vi "OLA.vi"() -> ()   [LabVIEW 2009]
doc: "This is the On-Line Analysis module (OLA).\nThis module receives events from the Target Event Builder (TEB) and processes them. The Q Curve is massaged, gains are divided out, the subtracted and poly subtracted signals are calculated, and an area measurement is made. These results are then sent to the Polarization Display Panel (PDP)."
uses:
  <vilib>/Analysis/NI_AALPro.lvlib
  <vilib>/Analysis/NI_AALBase.lvlib
panel:
  out "Bottom Charge":dbl format="%.6e"
  out "Top Charge":dbl format="%.6e"
  in  "Previous Event":i32
  in  "stop":bool
  out "RF Mod":i32
  out "RF Freq":dbl format="%.3f"
  out "Cal Const":dbl format="%.6f"
  out "Baseline":i32
  out "Raw Signal":dbl[](array[numeric]) format="%.4f"
  out "Event Number":i32
  out "Area":dbl format="%.6f"
  out "Polarization":dbl format="%.2f"
  out "PolySubtracted Signal":dbl[](array[numeric]) format="%.4f"
  out "Polyfit Curve":dbl[](array[numeric]) format="%.4f"
  out "Subtracted Signal":dbl[](array[numeric]) format="%.4f"
  out "Baseline Signal":dbl[](array[numeric]) format="%.6f"
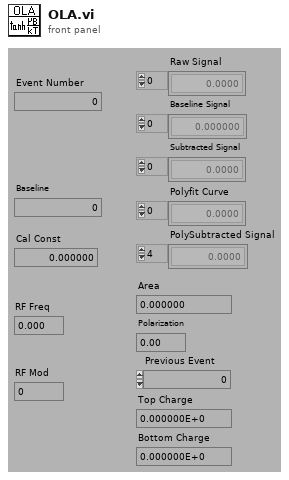
[diagram p1: front panel]
types:
  T1 = enum32{"SVD", "Givens", "Givens2", "Householder", "LU Decomposition", "Cholesky"}
  T2 = enum16{"No Message", "Bad Message", "ClearCharge", "Event=", "Address=", "Ping=", "Stop"}
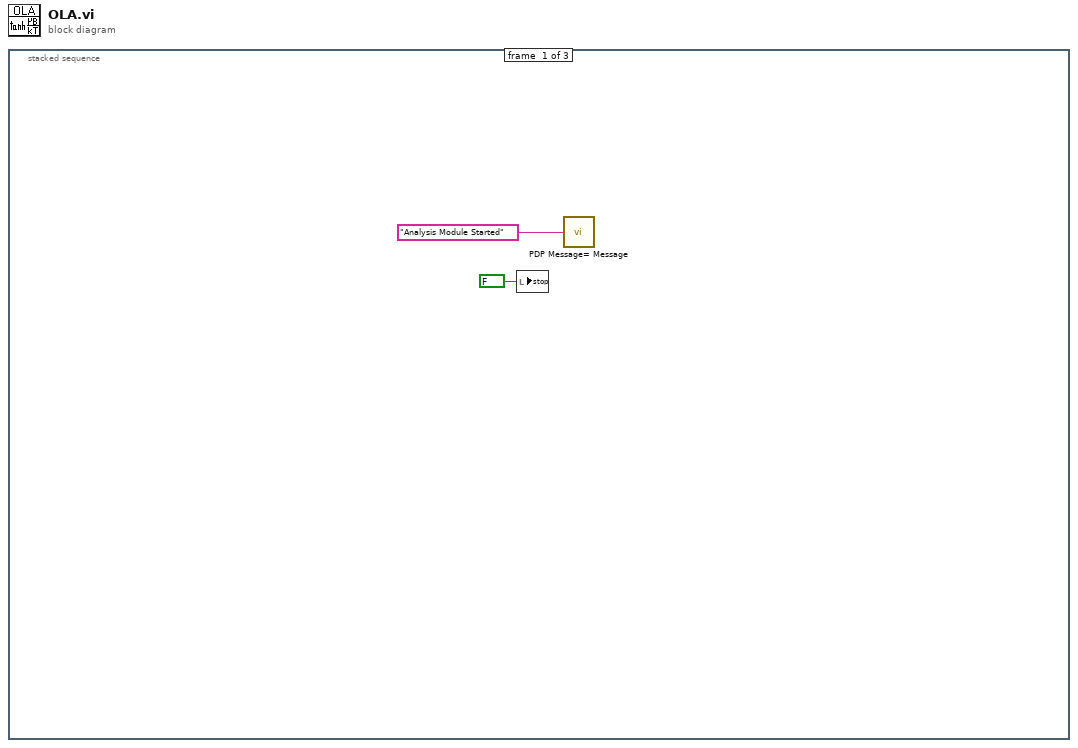
[diagram p0: block diagram]
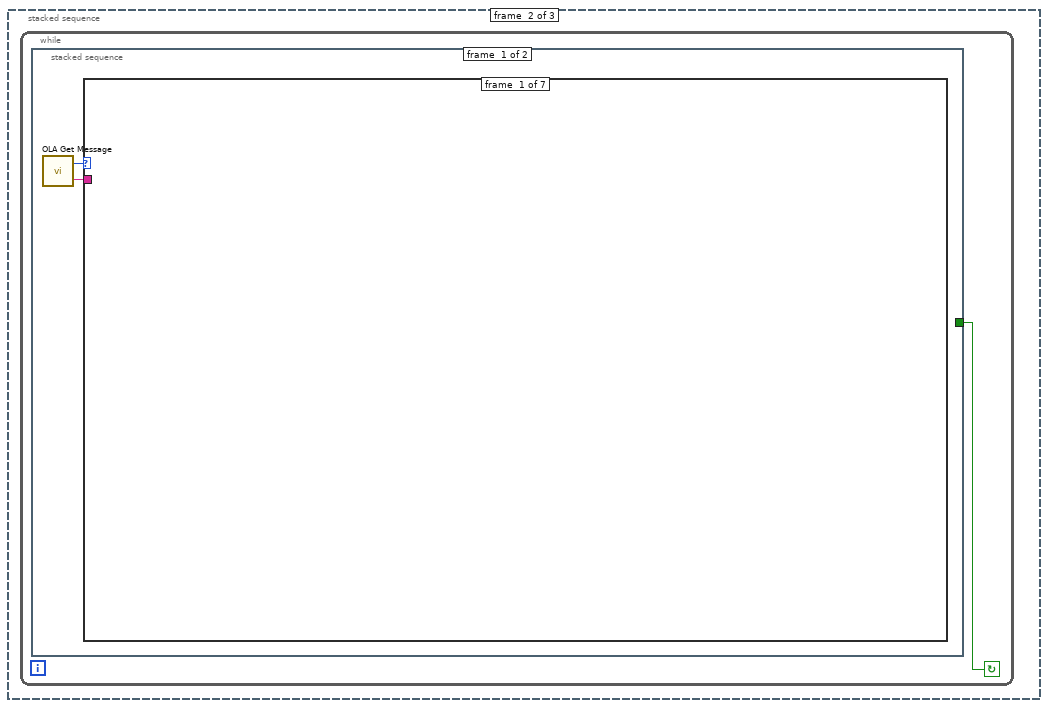
[diagram p2: hidden frame]
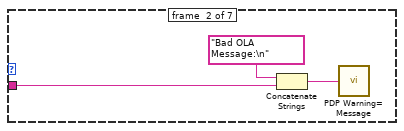
[diagram p3: hidden frame]
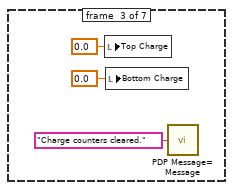
[diagram p4: hidden frame]
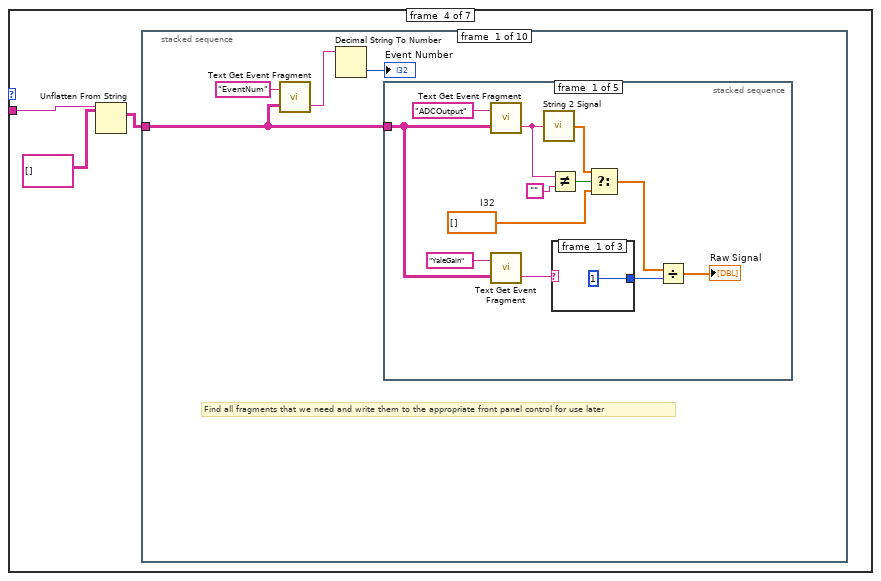
[diagram p5: hidden frame]
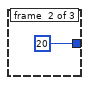
[diagram p6: hidden frame]
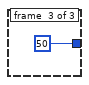
[diagram p7: hidden frame]
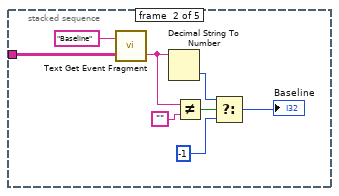
[diagram p8: hidden frame]
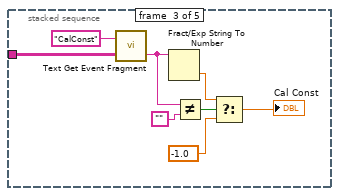
[diagram p9: hidden frame]
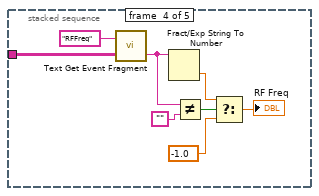
[diagram p10: hidden frame]
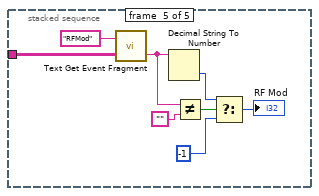
[diagram p11: hidden frame]
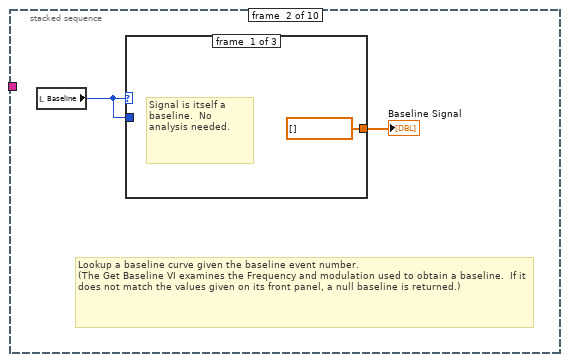
[diagram p12: hidden frame]
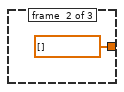
[diagram p13: hidden frame]
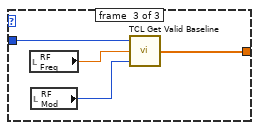
[diagram p14: hidden frame]
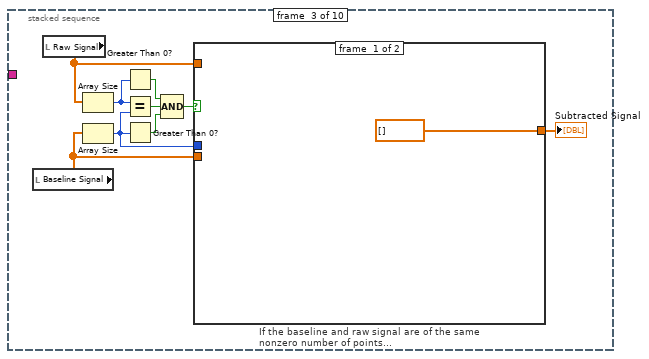
[diagram p15: hidden frame]
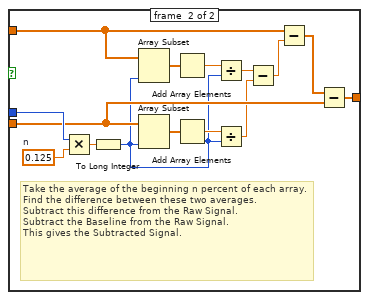
[diagram p16: hidden frame]
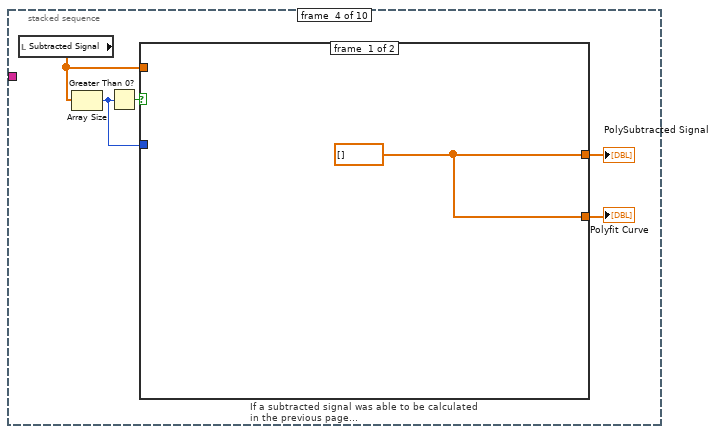
[diagram p17: hidden frame]
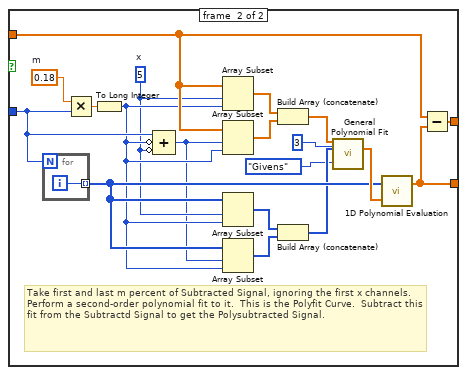
[diagram p18: hidden frame]
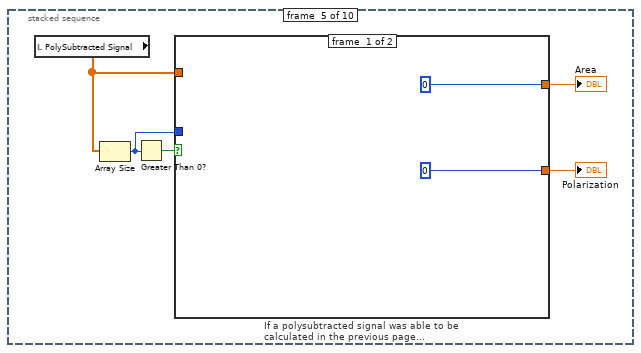
[diagram p19: hidden frame]
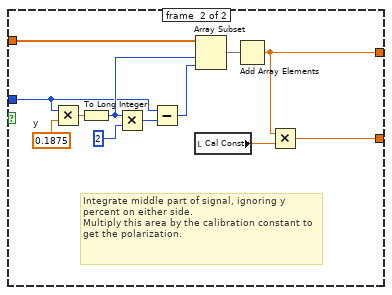
[diagram p20: hidden frame]
diagram:
  n1 = stacked-sequence {
    frame #0 {
      n2 = local write "stop"(FALSE ("stop")) -> ()
      n3 = call "PDP Message= Message.vi"("Message"="Analysis Module Started") -> ()
    }
    frame #1 {
      n4 = while {
        stop <- w3 continue-if-true
        n5 = stacked-sequence {
          tunnel: [_ w282] -> w3
          frame #0 {
            n6 = call "OLA Get Message.vi"() -> ("Text"=w5:string, "OLA Message Type"=w4:T2)
            n7 = case shown="\"Event=\"" w4 {
              tunnel: w5 -> [_ w8 _ w13 w274 w277 _]
              frame #0 {
              }
              frame #1 {
                n8 = Concatenate Strings("Bad OLA Message:\n", w8) -> (w6:string)
                n9 = call "PDP Warning= Message.vi"("Message"=w6) -> ()
              }
              frame #2 {
                n10 = local write "Top Charge"(0.0 ("Top Charge")) -> ()
                n11 = local write "Bottom Charge"(0.0 ("Bottom Charge")) -> ()
                n12 = call "PDP Message= Message.vi"("Message"="Charge counters cleared.") -> ()
              }
              frame #3 {
                (unwired) FALSE
                n13 = Unflatten From String(type=string[][] [], binary string=w13) -> (value=w12:string[][])  [unwired: 3 in, 2 out]
                n14 = stacked-sequence {
                  tunnel: w12 -> [w15 _ _ _ _ w147 w180 w199 _ _]
                  frame #0 {
                    # "Find all fragments that we need and write them to the appropriate front panel control for use later"
                    n15 = call "Text Get Event Fragment.vi"("Event"=w15, "Fragment Type"="EventNum") -> ("Fragment"=w17:string)  [unwired: 1 out]
                    n16 = Decimal String To Number(string=w17) -> (number=→"Event Number":i32)  [unwired: 2 in, 1 out]
                    n17 = stacked-sequence {
                      tunnel: w15 -> [w24 w40 w48 w56 w64]
                      frame #0 {
                        w19 = dbl[] []  # I32
                        n18 = call "Text Get Event Fragment.vi"("Event"=w24, "Fragment Type"="ADCOutput") -> ("Fragment"=w29:string)  [unwired: 1 out]
                        n19 = call "Text Get Event Fragment.vi"("Event"=w24, "Fragment Type"="YaleGain") -> ("Fragment"=w23:string)  [unwired: 1 out]
                        n20 = call "String 2 Signal.vi"("String"=w29) -> ("Signal"=w26:dbl[])
                        n21 = Not Equal?(x=w29, y="") -> (x != y?=w28:bool)
                        n22 = case shown="\"2\"" w23 {
                          tunnel: [1 20 50] -> w22
                          frame #0 {
                          }
                          frame #1 {
                          }
                          frame #2 {
                          }
                        }
                        n23 = Select(t=w26, s=w28, f=w19) -> (s? t:f=w21:dbl[])
                        n24 = Divide(x=w21, y=w22) -> (x/y=→"Raw Signal":dbl[])
                      }
                      frame #1 {
                        n25 = call "Text Get Event Fragment.vi"("Event"=w40, "Fragment Type"="Baseline") -> ("Fragment"=w35:string)  [unwired: 1 out]
                        n26 = Decimal String To Number(string=w35) -> (number=w38:i32)  [unwired: 2 in, 1 out]
                        n27 = Not Equal?(x=w35, y="") -> (x != y?=w37:bool)
                        n28 = Select(t=w38, s=w37, f=-1) -> (s? t:f=→"Baseline":i32)
                      }
                      frame #2 {
                        n29 = call "Text Get Event Fragment.vi"("Event"=w48, "Fragment Type"="CalConst") -> ("Fragment"=w43:string)  [unwired: 1 out]
                        n30 = Fract/Exp String To Number(string=w43) -> (number=w46:dbl)  [unwired: 3 in, 1 out]
                        n31 = Not Equal?(x=w43, y="") -> (x != y?=w45:bool)
                        n32 = Select(t=w46, s=w45, f=-1.0) -> (s? t:f=→"Cal Const":dbl)
                      }
                      frame #3 {
                        n33 = call "Text Get Event Fragment.vi"("Event"=w56, "Fragment Type"="RFFreq") -> ("Fragment"=w51:string)  [unwired: 1 out]
                        n34 = Fract/Exp String To Number(string=w51) -> (number=w54:dbl)  [unwired: 3 in, 1 out]
                        n35 = Not Equal?(x=w51, y="") -> (x != y?=w53:bool)
                        n36 = Select(t=w54, s=w53, f=-1.0) -> (s? t:f=→"RF Freq":dbl)
                      }
                      frame #4 {
                        n37 = call "Text Get Event Fragment.vi"("Event"=w64, "Fragment Type"="RFMod") -> ("Fragment"=w59:string)  [unwired: 1 out]
                        n38 = Decimal String To Number(string=w59) -> (number=w62:i32)  [unwired: 2 in, 1 out]
                        n39 = Not Equal?(x=w59, y="") -> (x != y?=w61:bool)
                        n40 = Select(t=w62, s=w61, f=-1) -> (s? t:f=→"RF Mod":i32)
                      }
                    }
                  }
                  frame #1 {
                    # "Lookup a baseline curve given the baseline event number.\n(The Get Baseline VI examines the Frequency and modulation used to obtain a baseline.  If it does not match the values given on its front panel, a null baseline is returned.)"
                    n41 = local read "Baseline"() -> (w67:i32)
                    n42 = case shown="1, Default" w67 {
                      tunnel: w67 -> [_ _ w73]
                      tunnel: [dbl[] [] ("Baseline") dbl[] [] ("Baseline") w70] -> w66
                      frame #0 {
                        # "Signal is itself a baseline.  No analysis needed."
                      }
                      frame #1 {
                      }
                      frame #2 {
                        n43 = local read "RF Freq"() -> (w72:dbl)
                        n44 = local read "RF Mod"() -> (w71:i32)
                        n45 = call "TCL Get Valid Baseline.vi"("RFMod (kHz)"=w71, "RFFreq (MHz)"=w72, "Baseline Event #"=w73) -> ("Baseline"=w70:dbl[])
                      }
                    }
                    "Baseline Signal" <- w66
                  }
                  frame #2 {
                    n46 = local read "Baseline Signal"() -> (w82:dbl[])
                    n47 = local read "Raw Signal"() -> (w81:dbl[])
                    n48 = Array Size(array=w81) -> (size(s)=w79:i32)
                    n49 = Array Size(array=w82) -> (size(s)=w80:i32)
                    n50 = Greater Than 0?(x=w79) -> (x > 0?=w76:bool)
                    n51 = Equal?(x=w79, y=w80) -> (x = y?=w77:bool)
                    n52 = Greater Than 0?(x=w80) -> (x > 0?=w78:bool)
                    n53 = Compound Arithmetic op=AND(w76, w77, w78) -> (w75:bool)
                    n54 = case "If the baseline and raw signal are of the same nonzero number of points..." shown="True" w75 {
                      tunnel: w82 -> [_ w91]
                      tunnel: w81 -> [_ w93]
                      tunnel: w80 -> [_ w98]
                      tunnel: [dbl[] [] w84] -> w74
                      frame #0 {
                      }
                      frame #1 {
                        w96 = 0.125  # n
                        # "Take the average of the beginning n percent of each array.\nFind the difference between these two averages.\nSubtract this difference from the Raw Signal.\nSubtract the Baseline from the Raw Signal.\nThis gives the Subtracted Signal."
                        n55 = Multiply(x=w98, y=w96) -> (x*y=w97:dbl)
                        n56 = To Long Integer(number=w97) -> (32bit integer=w85:i32)
                        n57 = Array Subset(array=w93, length=w85) -> (w95:dbl[])  [unwired: 1 in]
                        n58 = Array Subset(array=w91, length=w85) -> (w94:dbl[])  [unwired: 1 in]
                        n59 = Add Array Elements(numeric array=w95) -> (sum=w89:dbl)
                        n60 = Add Array Elements(numeric array=w94) -> (sum=w90:dbl)
                        n61 = Divide(x=w89, y=w85) -> (x/y=w88:dbl)
                        n62 = Divide(x=w90, y=w85) -> (x/y=w87:dbl)
                        n63 = Subtract(x=w88, y=w87) -> (x-y=w86:dbl)
                        n64 = Subtract(x=w93, y=w86) -> (x-y=w92:dbl[])
                        n65 = Subtract(x=w92, y=w91) -> (x-y=w84:dbl[])
                      }
                    }
                    "Subtracted Signal" <- w74
                  }
                  frame #3 {
                    n66 = local read "Subtracted Signal"() -> (w101:dbl[])
                    n67 = Array Size(array=w101) -> (size(s)=w102:i32)
                    n68 = Greater Than 0?(x=w102) -> (x > 0?=w103:bool)
                    n69 = case "If a subtracted signal was able to be calculated in the previous page..." shown="True" w103 {
                      tunnel: w102 -> [_ w108]
                      tunnel: w101 -> [_ w111]
                      tunnel: [w104 w110] -> w100
                      tunnel: [w104 w109] -> w99
                      frame #0 {
                        w104 = dbl[] []
                      }
                      frame #1 {
                        w106 = 5  # x
                        w123 = 0.18  # m
                        # "Take first and last m percent of Subtracted Signal, ignoring the first x channels.  Perform a second-order polynomial fit to it.  This is the Polyfit Curve.  Subtract this fit from the Subtractd Signal to get the Polysubtracted Signal."
                        n70 = for {
                          N: w108 -> [_]
                          tunnel: [w124] -> w116 mode=indexing
                          i -> [w124]
                        }
                        n71 = Multiply(x=w123, y=w108) -> (x*y=w122:dbl)
                        n72 = To Long Integer(number=w122) -> (32bit integer=w107:i32)
                        n73 = Compound Arithmetic op=ADD(w108, invert w107, invert w106) -> (w105:i32)
                        n74 = Array Subset(array=w111, index=w106, length=w107) -> (w121:dbl[])
                        n75 = Array Subset(array=w111, index=w105, length=w107) -> (w120:dbl[])
                        n76 = Array Subset(array=w116, index=w106, length=w107) -> (w119:i32[])
                        n77 = Array Subset(array=w116, index=w105, length=w107) -> (w118:i32[])
                        n78 = Build Array (concatenate)(w121, w120) -> (w115:dbl[])
                        n79 = Build Array (concatenate)(w119, w118) -> (w114:i32[])
                        n80 = call <vilib>:"General Polynomial Fit.vi"("Y"=w115, "polynomial order"=3, "X"=w114, "algorithm"=T1."Givens") -> ("Polynomial Coefficients"=w117:dbl[])  [unwired: 8 in, 3 out]
                        n81 = call <vilib>:"1D Polynomial Evaluation.vi"("Coefficients: a"=w117, "X"=w116) -> ("Y"=w109:dbl[])  [unwired: 1 out]
                        n82 = Subtract(x=w111, y=w109) -> (x-y=w110:dbl[])
                      }
                    }
                    "Polyfit Curve" <- w99
                    "PolySubtracted Signal" <- w100
                  }
                  frame #4 {
                    n83 = local read "PolySubtracted Signal"() -> (w128:dbl[])
                    n84 = Array Size(array=w128) -> (size(s)=w127:i32)
                    n85 = Greater Than 0?(x=w127) -> (x > 0?=w129:bool)
                    n86 = case "If a polysubtracted signal was able to be calculated in the previous page..." shown="True" w129 {
                      tunnel: w128 -> [_ w143]
                      tunnel: w127 -> [_ w135]
                      tunnel: [0 w134] -> w126
                      tunnel: [0 w133] -> w125
                      frame #0 {
                      }
                      frame #1 {
                        w141 = 0.1875  # y
                        # "Integrate middle part of signal, ignoring y percent on either side.\nMultiply this area by the calibration constant to get the polarization."
                        n87 = Multiply(x=w135, y=w141) -> (x*y=w139:dbl)
                        n88 = To Long Integer(number=w139) -> (32bit integer=w136:i32)
                        n89 = Multiply(x=w136, y=2) -> (x*y=w137:i32)
                        n90 = Subtract(x=w135, y=w137) -> (x-y=w140:i32)
                        n91 = local read "Cal Const"() -> (w132:dbl)
                        n92 = Array Subset(array=w143, index=w136, length=w140) -> (w142:dbl[])
                        n93 = Add Array Elements(numeric array=w142) -> (sum=w134:dbl)
                        n94 = Multiply(x=w134, y=w132) -> (x*y=w133:dbl)
                      }
                    }
                    "Polarization" <- w125
                    "Area" <- w126
                  }
                  frame #5 {
                    n95 = call "Text Get Event Fragment.vi"("Event"=w147, "Fragment Type"="ptpos") -> ("Fragment"=w145:string)  [unwired: 1 out]
                    n96 = call "Text Get Event Fragment.vi"("Event"=w147, "Fragment Type"="ibcm2") -> ("Fragment"=w156:string, "Found"=w144:bool)
                    n97 = call "Text Get Event Fragment.vi"("Event"=w147, "Fragment Type"="LL91112") -> ("Fragment"=w158:string)  [unwired: 1 out]
                    n98 = Fract/Exp String To Number(string=w156) -> (number=w155:dbl)  [unwired: 3 in, 1 out]
                    n99 = Fract/Exp String To Number(string=w158) -> (number=w157:dbl)  [unwired: 3 in, 1 out]
                    n100 = Greater?(x=w155, y=20.0) -> (0:w150:bool)
                    n101 = Less?(x=w155, y=200.0) -> (x < y?=w152:bool)
                    n102 = Not Equal To 0?(x=w157) -> (x != 0?=w151:bool)
                    n103 = Compound Arithmetic op=AND(w144, w150, w152, w151) -> (w149:bool)
                    n104 = case shown="True" w149 {
                      tunnel: w155 -> [_ w170]
                      tunnel: w145 -> [_ w161]
                      frame #0 {
                      }
                      frame #1 {
                        w169 = 100  # n
                        # "Only add to charge if less than n seconds since last event"
                        n105 = local read "Event Number"() -> (w160:i32)
                        n106 = Subtract(x=w160, y="Previous Event") -> (x-y=w166:i32)
                        n107 = case shown="\"1\"" w161 {
                          tunnel: [0.0 w177 w178] -> w163
                          frame #0 {
                          }
                          frame #1 {
                            n108 = local read "Top Charge"() -> (w177:dbl)
                          }
                          frame #2 {
                            n109 = local read "Bottom Charge"() -> (w178:dbl)
                          }
                        }
                        n110 = Less?(x=w166, y=w169) -> (x < y?=w167:bool)
                        n111 = Select(t=w166, s=w167, f=0) -> (s? t:f=w164:i32)
                        n112 = Compound Arithmetic op=MULTIPLY(w170, 6.241418050181001e+18, 1e-09 ("Input"), w164) -> (w168:dbl)
                        n113 = Add(x=w163, y=w168) -> (x+y=w162:dbl)
                        n114 = local write "Previous Event"(w160) -> ()
                        n115 = case shown="\"1\"" w161 {
                          tunnel: w162 -> [_ w174 w175]
                          frame #0 {
                          }
                          frame #1 {
                            "Top Charge" <- w174
                          }
                          frame #2 {
                            "Bottom Charge" <- w175
                          }
                        }
                      }
                    }
                  }
                  frame #6 {
                    n116 = call "Text Get Event Fragment.vi"("Event"=w180, "Fragment Type"="He4Temp") -> ("Found"=w179:bool)  [unwired: 1 out]
                    n117 = case shown="False" w179 {
                      tunnel: w180 -> [w188 _]
                      frame #0 {
                        n118 = call "Text Get Event Fragment.vi"("Event"=w188, "Fragment Type"="He4Press") -> ("Fragment"=w196:string)  [unwired: 1 out]
                        n119 = call "Text Get Event Fragment.vi"("Event"=w188, "Fragment Type"="He4Range") -> ("Fragment"=w187:string)  [unwired: 1 out]
                        n120 = Fract/Exp String To Number(string=w196) -> (number=w182:dbl)  [unwired: 3 in, 1 out]
                        n121 = Fract/Exp String To Number(string=w187) -> (number=w186:dbl)  [unwired: 3 in, 1 out]
                        n122 = expression code="10**(-x+2)"(w186) -> (w185:dbl)
                        n123 = Multiply(x=w182, y=w185) -> (x*y=w183:dbl)
                        n124 = call "TTM 4He Press to Temp.vi"("4He Vapor Pressure (torr)"=w183) -> ("4He Temp (K)"=w184:dbl)
                        n125 = Number To Exponential String(number=w184) -> (E-format string=w194:string)  [unwired: 3 in]
                        n126 = local read "Event Number"() -> (w191:i32)
                        n127 = Build Array("He4Temp", w194) -> (w190:string[])
                        n128 = Build Array(w190) -> (w192:string[][])
                        n129 = call "TEB EventFrag= Message.vi"("Event Fragment(s)"=w192, "Event Number"=w191) -> ()
                      }
                      frame #1 {
                      }
                    }
                  }
                  frame #7 {
                    n130 = call "Text Get Event Fragment.vi"("Event"=w199, "Fragment Type"="HPFreq") -> ("Fragment"=w197:string, "Found"=w198:bool)
                    n131 = case shown="True" w198 {
                      tunnel: w199 -> [w202 w220]
                      tunnel: w197 -> [_ w217]
                      frame #0 {
                        n132 = call "Text Get Event Fragment.vi"("Event"=w202, "Fragment Type"="EIPFreq") -> ("Fragment"=w201:string)  [unwired: 1 out]
                        n133 = local read "Event Number"() -> (w204:i32)
                        n134 = Build Array("uWaveFreq", w201) -> (w203:string[])
                        n135 = Build Array(w203) -> (w205:string[][])
                        n136 = call "TEB EventFrag= Message.vi"("Event Fragment(s)"=w205, "Event Number"=w204) -> ()
                      }
                      frame #1 {
                        n137 = call "Text Get Event Fragment.vi"("Event"=w220, "Fragment Type"="EIPFreq") -> ("Fragment"=w219:string)  [unwired: 1 out]
                        n138 = Fract/Exp String To Number(string=w217) -> (number=w210:dbl)  [unwired: 3 in, 1 out]
                        n139 = Fract/Exp String To Number(string=w219) -> (number=w218:dbl)  [unwired: 3 in, 1 out]
                        n140 = Multiply(x=w218, y=2) -> (x*y=w216:dbl)
                        n141 = Add(x=w210, y=w216) -> (x+y=w215:dbl)
                        n142 = Equal To 0?(x=w210) -> (x = 0?=w209:bool)
                        n143 = Number To Fractional String(number=w215, precision (6)=i16 3) -> (F-format string=w211:string)  [unwired: 2 in]
                        n144 = Select(t="0", s=w209, f=w211) -> (s? t:f=w212:string)
                        n145 = local read "Event Number"() -> (w222:i32)
                        n146 = Build Array("uWaveFreq", w212) -> (w221:string[])
                        n147 = Build Array(w221) -> (w223:string[][])
                        n148 = call "TEB EventFrag= Message.vi"("Event Fragment(s)"=w223, "Event Number"=w222) -> ()
                      }
                    }
                  }
                  frame #8 {
                    w228 = string[] [] ("Array Constant")
                    # "Ship all results off to the event builder."
                    n149 = local read "PolySubtracted Signal"() -> (w226:dbl[])
                    n150 = local read "Polyfit Curve"() -> (w262:dbl[])
                    n151 = local read "Bottom Charge"() -> (w238:dbl)
                    n152 = local read "Subtracted Signal"() -> (w263:dbl[])
                    n153 = local read "Top Charge"() -> (w239:dbl)
                    n154 = local read "Polarization"() -> (w249:dbl)
                    n155 = local read "Raw Signal"() -> (w246:dbl[])
                    n156 = local read "Baseline Signal"() -> (w268:dbl[])
                    n157 = local read "Area"() -> (w257:dbl)
                    n158 = Array Size(array=w226) -> (size(s)=w227:i32)
                    n159 = Equal To 0?(x=w227) -> (x = 0?=w229:bool)
                    n160 = call "Signal 2 String.vi"("Signal"=w246) -> ("String"=w247:string)
                    n161 = call "Signal 2 String.vi"("Signal"=w268) -> ("String"=w267:string)
                    n162 = call "Signal 2 String.vi"("Signal"=w263) -> ("String"=w264:string)
                    n163 = call "Signal 2 String.vi"("Signal"=w262) -> ("String"=w261:string)
                    n164 = call "Signal 2 String.vi"("Signal"=w226) -> ("String"=w258:string)
                    n165 = Number To Exponential String(number=w239) -> (E-format string=w241:string)  [unwired: 3 in]
                    n166 = Number To Exponential String(number=w238) -> (E-format string=w236:string)  [unwired: 3 in]
                    n167 = Number To Exponential String(number=w249) -> (E-format string=w250:string)  [unwired: 3 in]
                    n168 = Number To Exponential String(number=w257) -> (E-format string=w256:string)  [unwired: 3 in]
                    n169 = Build Array("RawSignal", w247) -> (w245:string[])
                    n170 = Build Array("BaseSignal", w267) -> (w244:string[])
                    n171 = Build Array("SubSignal", w264) -> (w243:string[])
                    n172 = Build Array("PolyCurve", w261) -> (w242:string[])
                    n173 = Build Array("PolySignal", w258) -> (w254:string[])
                    n174 = Build Array("TopCharge", w241) -> (w235:string[])
                    n175 = Build Array("BottomCharge", w236) -> (w234:string[])
                    n176 = Build Array("Polarization", w250) -> (w233:string[])
                    n177 = Build Array("Area", w256) -> (w232:string[])
                    n178 = Select(t=w228, s=w229, f=w233) -> (s? t:f=w230:string[])
                    n179 = Select(t=w228, s=w229, f=w232) -> (s? t:f=w231:string[])
                    n180 = local read "Event Number"() -> (w252:i32)
                    n181 = Build Array(w245, w244, w243, w242, w254, w235, w234, w230, w231) -> (w253:string[][])
                    n182 = call "TEB EventFrag= Message.vi"("Event Fragment(s)"=w253, "Event Number"=w252) -> ()
                  }
                  frame #9 {
                    # "Tell event builder we're done processing this event."
                    n183 = local read "Event Number"() -> (w270:i32)
                    n184 = call "TEB Processed= Message.vi"("Module Name"="OLA", "Event Number"=w270) -> ()
                  }
                }
              }
              frame #4 {
                n185 = Scan From String(format string="%s,%[.0-9]:%d" ("Format String"), input string=w274) -> (output 1=w272:string, output 2=w273:string, output 3=w271:i32)  [unwired: 5 in, 3 out]
                n186 = call "Message Set Module Address.vi"("Port"=w271, "Address"=w273, "Module"=w272) -> ()
              }
              frame #5 {
                n187 = Get Date/Time In Seconds() -> (seconds since 1Jan1904=w276:timestamp)
                n188 = To Double Precision Float(number=w276) -> (double precision float=w279:dbl)
                n189 = Format Into String(format string="PingResponse=OLA,%.0f", w279) -> (resulting string=w278:string)  [unwired: 2 in, 1 out]
                n190 = call "Message Send.vi"("Message"=w278, "Destination"=w277) -> ()
              }
              frame #6 {
                n191 = local write "stop"(TRUE ("stop")) -> ()
              }
            }
          }
          frame #1 {
            n192 = Not(x="stop") -> (.not. x?=w282:bool)
          }
        }
      }
    }
    frame #2 {
      n193 = local write "stop"(FALSE ("stop")) -> ()
      n194 = call "PDP Message= Message.vi"("Message"="OLA Module Stopped") -> ()
    }
  }
